vi "MessageTableProbe.vi"(1 "Message":refnum<class "MSG.lvclass">) -> (0 "Boolean":bool)   [LabVIEW 2011, in "Messenging.lvlib"]
uses:
  Messenging.lvlib
  Interprocess Messenger/TextVarientMessage/MSG.lvclass
  Interprocess Messenger/Send/Send.lvclass
panel:
  out "Table":string[][](table)
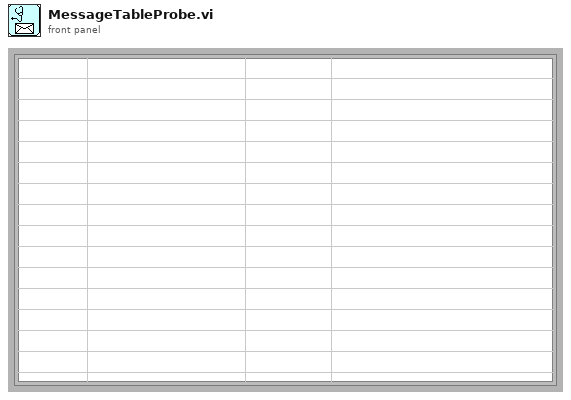
[diagram p1: front panel]
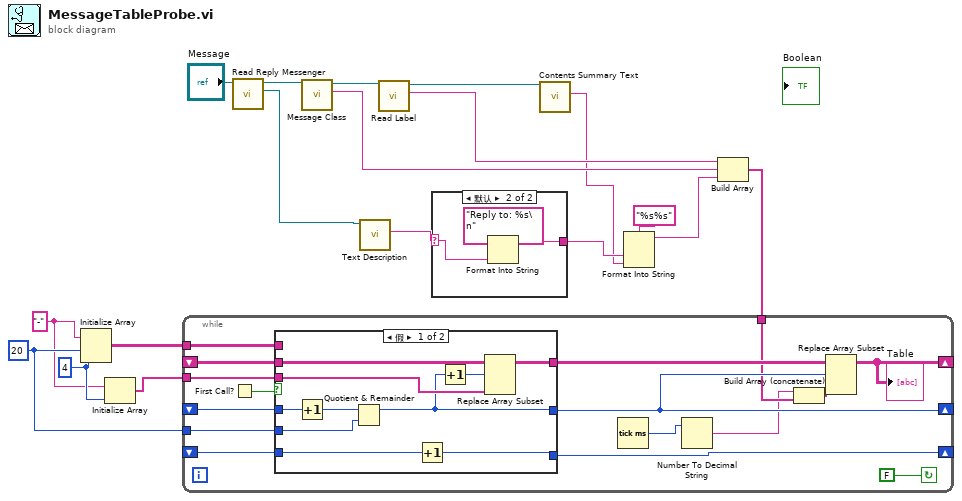
[diagram p0: block diagram]
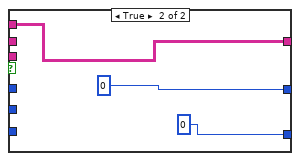
[diagram p2: hidden frame]
diagram:
  w2 = "-" ("Message Class")
  w3 = 4 ("dimension size")
  w4 = 20 ("dimension size")
  n1 = Initialize Array(w2, w4, w3) -> (w5:string[][])
  n2 = Initialize Array(w2, w3) -> (w1:string[])
  n3 = call-dynamic "Read Reply Messenger.vi"("Messege"="Message") -> ("Reply to..."=w8:refnum<class "Send.lvclass">, "Message"=w13:refnum<class "MSG.lvclass">)  [unwired: 1 in, 8 out]
  n4 = call-dynamic "Message Class.vi"("Message"=w13) -> ("Message Class"=w15:string, "Message"=w18:refnum<class "MSG.lvclass">)  [unwired: 1 in, 8 out]
  n5 = call-dynamic "Text Description.vi"("Send in"=w8) -> ("Description"=w7:string)  [unwired: 10 out]
  n6 = call-dynamic "Read Label.vi"("Message"=w18) -> ("Label"=w16:string, "Message"=w17:refnum<class "MSG.lvclass">)  [unwired: 1 in, 8 out]
  n7 = case shown="默认" w7 {
    selector: w7 -> [w19 w20]
    tunnel: [w19 w22] -> w11
    frame "" {
    }
    frame Default {
      n8 = Format Into String(format string="Reply to: %s\n", w20) -> (resulting string=w22:string)  [unwired: 2 in, 1 out]
    }
  }
  n9 = call-dynamic "Contents Summary Text.vi"("Message"=w17) -> ("Contents Summary Text"=w10:string)  [unwired: 10 out]
  n10 = Format Into String(format string="%s%s", w11, w10) -> (resulting string=w9:string)  [unwired: 2 in, 1 out]
  n11 = Build Array(w16, w15, w9) -> (w6:string[])
  n12 = while {
    tunnel: w6 -> [w27]
    shift-right: [w32] -> _
    shift-left: _ -> [w36]
    shift-right: [w33] -> _
    shift-left: _ -> [w35]
    tunnel: w5 -> [w30]
    tunnel: w4 -> [w34]
    tunnel: w1 -> [w29]
    shift-right: [w26] -> _
    shift-left: _ -> [w25]
    stop <- FALSE continue-if-true
    n13 = First Call?() -> (First Call?: T/F=w38:bool)
    n14 = case shown="假" w38 {
      tunnel: [w44 w50] -> w37
      tunnel: w36 -> [w45 _]
      tunnel: [w41 0 ("index (row)")] -> w33
      tunnel: w35 -> [w48 _]
      tunnel: w34 -> [w46 _]
      tunnel: w30 -> [_ w50]
      tunnel: w29 -> [w43 _]
      tunnel: [w39 0 ("index (row)")] -> w26
      tunnel: w25 -> [w40 _]
      frame False {
        n15 = Increment(x=w48) -> (x+1=w47:i32)
        n16 = Quotient & Remainder(x=w47, y=w46) -> (x-y*floor(x/y)=w41:i32)  [unwired: 1 out]
        n17 = Increment(x=w40) -> (x+1=w39:i32)
        n18 = Increment(x=w41) -> (x+1=w42:i32)
        n19 = Replace Array Subset(array=w45, new element=w43, index (row)=w42) -> (w44:string[][])  [unwired: 1 in]
      }
      frame True {
      }
    }
    n20 = Tick Count (ms)() -> (millisecond timer value=w24:u32)
    n21 = Number To Decimal String(number=w24) -> (decimal integer string=w23:string)  [unwired: 1 out]
    n22 = Build Array (concatenate)(w23, w27) -> (w28:string[])
    n23 = Replace Array Subset(array=w37, new element=w28, index (row)=w33) -> (w32:string[][])  [unwired: 1 in]
    "Table" <- w32
  }
